vi "总磷总氮通讯.vi"() -> ()   [LabVIEW 2016, in "斯坦道总磷.lvlib"]
uses:
  <vilib>/NI/Modbus Library/API/Wrapper/Create TCP Slave.vi
  <vilib>/Utility/config.llb/Write Key (Boolean).vi
  <vilib>/Utility/config.llb/Write Key (String).vi
  <vilib>/Plasmionique/MB Master/MB_Master/MB_Master.lvclass
  <vilib>/NI/Modbus Library/API/Slave/Modbus Slave.lvclass
  <vilib>/Utility/config.llb/NI_LVConfig.lvlib
  <vilib>/Plasmionique/MB Master/MB Master.lvlib
  <vilib>/NI/Modbus Library/API/Wrapper/API Main.lvlib
  <vilib>/ptbypt/NI_PtbyPt.lvlib
panel:
  out "氨氮状态告警区":u16[](array[numeric])
  out "氨氮测量数据区":u16[](array[numeric])
  out "COD测量数据区":u16[](array[numeric])
  out "COD状态告警区":u16[](array[numeric])
  out "总氮测量数据区":u16[](array[numeric])
  out "总氮状态告警区":u16[](array[numeric])
  out "总磷状态告警区":u16[](array[numeric])
  out "总磷测量数据区":u16[](array[numeric])
  out "状态告警区":T1 {"告警代码" items=["无告警", "缺试剂告警", "缺水样告警", "缺蒸馏水告警", "缺标液告警", "仪表漏液告警", "标定异常告警", "超量程告警", "加热异常", "低试剂预警", "超上限告警", "超下限告警", "仪表内部其他异常", "滴定异常告警", "电极异常告警", "量程切换告警", "参数设置告警", "PH电极电位异常", "电导率电极异常", "浊度光度异常", "溶解氧电极异常", "溶解氧光强异常", "温度异常告警", "PH异常告警", "溶解氧异常告警", "电导率异常告警", "浊度异常告警", "叶绿素异常告警", "藻密度异常告警", "蓝绿藻异常告警", "ORP异常告警", "氨氮异常告警", "清洁刷异常告警", "SD卡异常告警", "蓝牙异常告警", "Wifi异常告警", "流程异常告警"]; "故障代码" items=["无故障", "电机故障", "温度故障", "通讯故障", "滴定故障"]}
  out "测量数据区":T2 {"单位" items=["ug/L", "mg/L", "ppm", "mg/m3", "cm", "ppb", "ug/m3", "%", "nmol/mol", "umol/mol", "MPN/L", "MPN/100ml", "ng/m3", "NTU", "无量纲", "ms/cm", "us/cm", "℃", "mV", "万个/L"]}
  out "status":bool
  out "关键参数区":T3
  in  "读关键参数区":bool
  in  "读状态告警区":bool
  in  "读测量数据区":bool
  in  "站号":u16(ring) items=["总磷"=1, "氨氮"=3]
  in  "停止":bool
  in  "启动":bool
  in  "控制命令":u16(ring) items=["启动测量"=1, "标样核查"=2, "零点核查"=3, "跨度核查"=4, "空白测试"=5, "平行样测试"=6, "加标回收"=7, "空白校准"=8, "标样校准"=9, "初始化（清洗）"=10, "停止测试"=11, "仪器重启"=12, "校时"=13, "模式设置"=14, "测量间隔设置"=15]
  in  "控制命令参数":u16[](array[numeric]) format="%04xH"
  in  "VISA Resource":refnum<visa-resource-name>
  in  "启用模块":bool
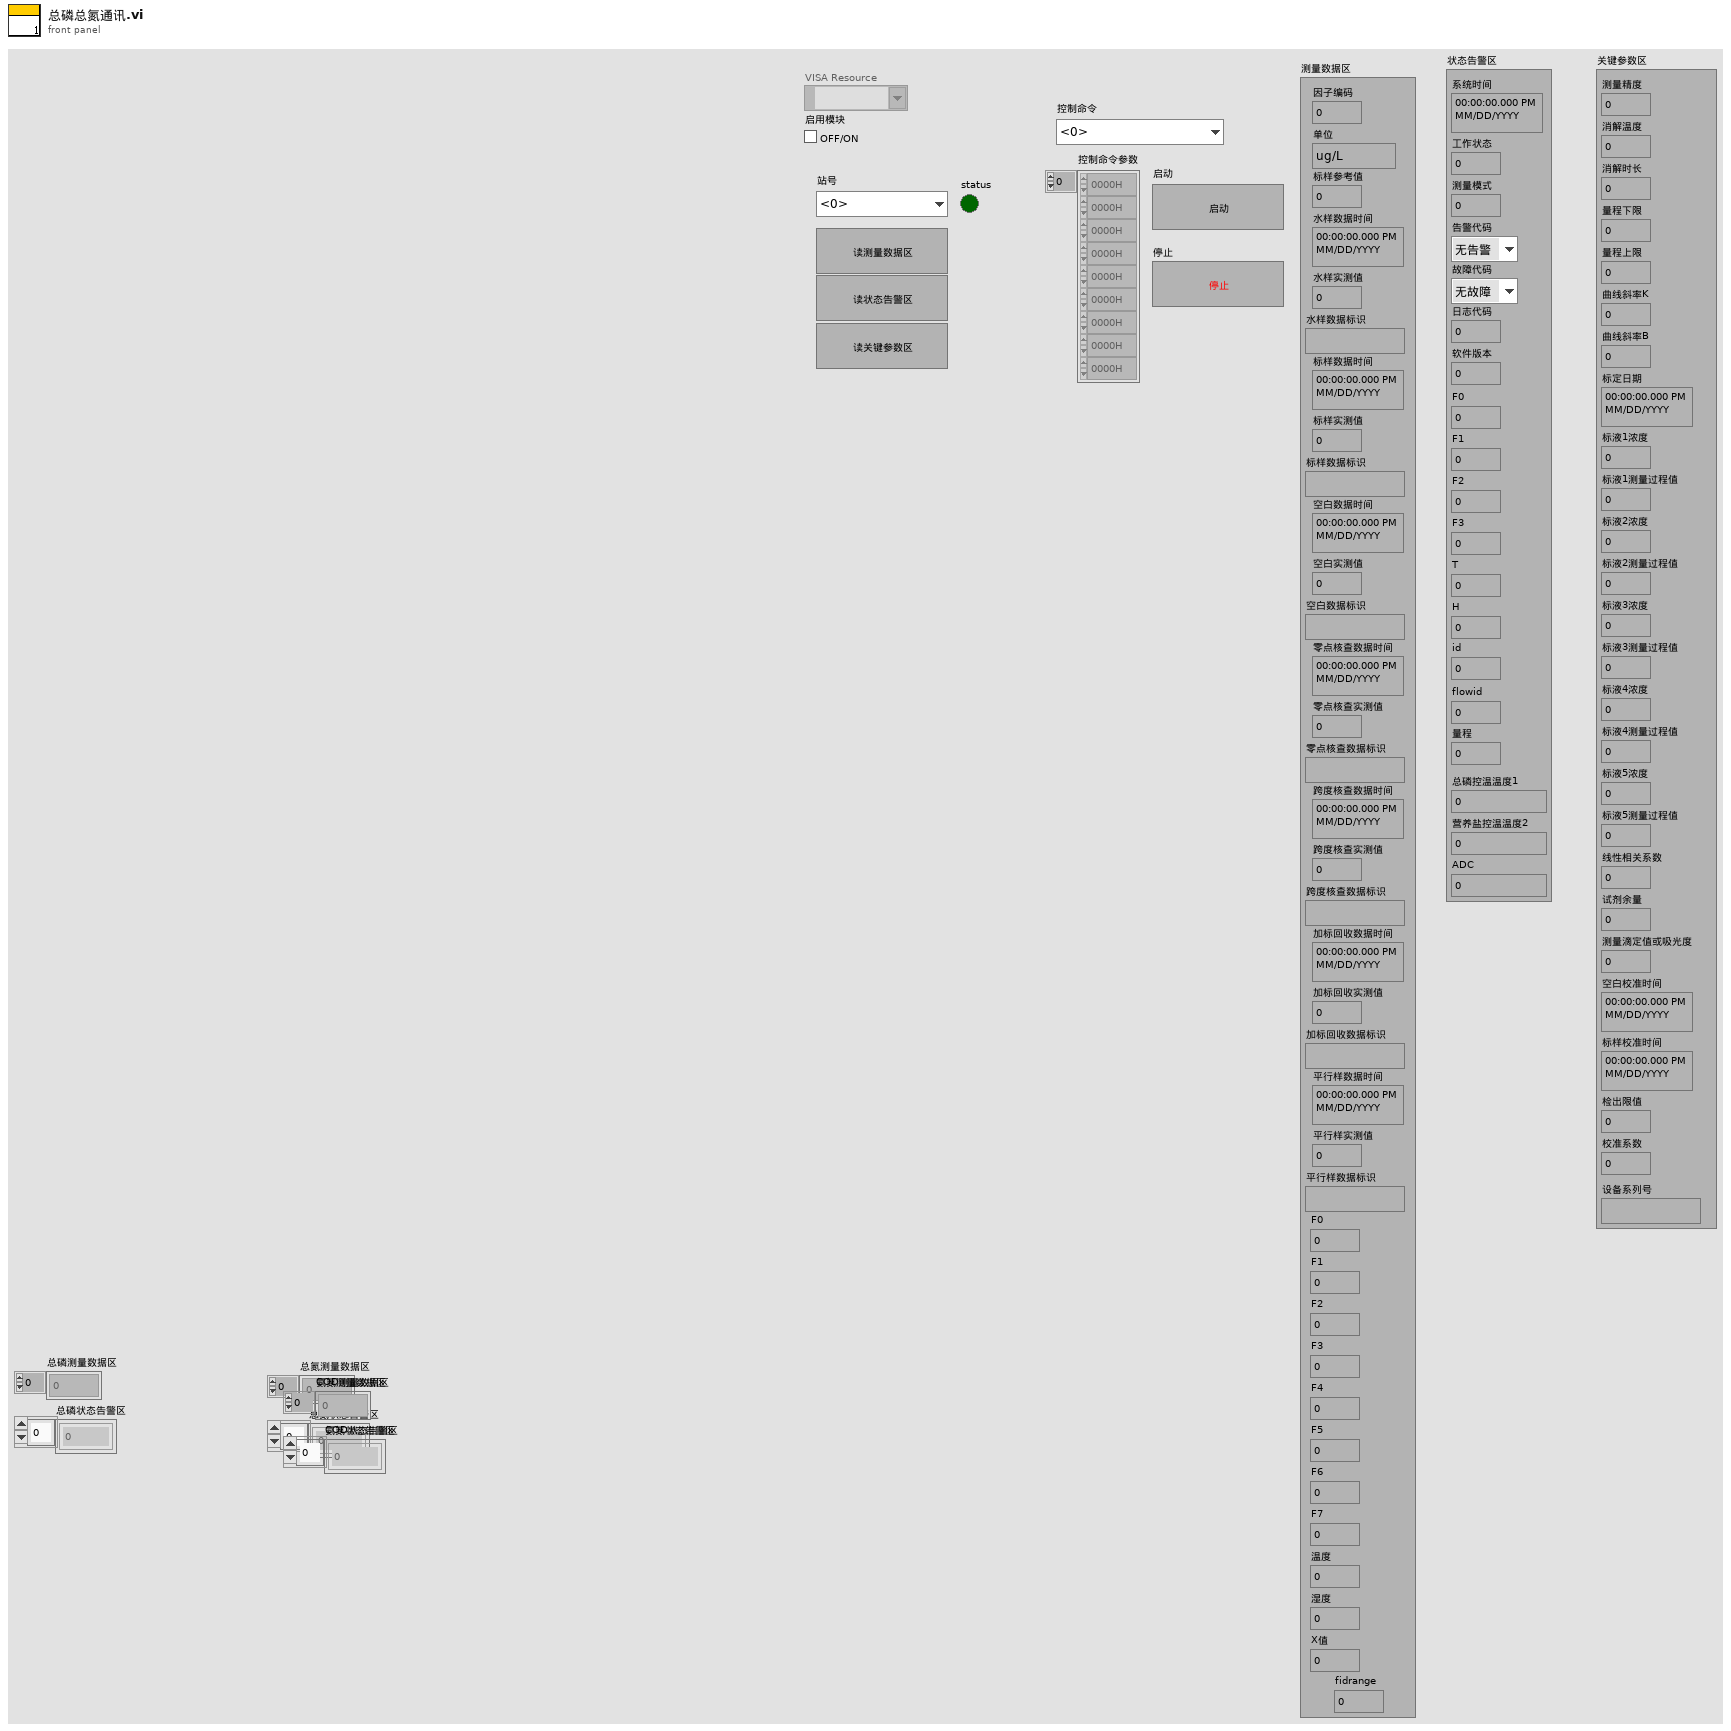
[diagram p1: front panel]
types:
  T1 = cluster{"系统时间":timestamp, "工作状态":u16, "测量模式":u16, "告警代码":u16, "故障代码":u16, "日志代码":u16, "软件版本":u16, "F0":sgl, "F1":sgl, "F2":sgl, "F3":sgl, "T":sgl, "H":sgl, "id":u16, "flowid":u16, "量程":u16, "总磷控温温度1":sgl, "营养盐控温温度2":sgl, "ADC":sgl}
  T2 = cluster{"因子编码":u32, "单位":u16, "标样参考值":sgl, "水样数据时间":timestamp, "水样实测值":sgl, "水样数据标识":string, "标样数据时间":timestamp, "标样实测值":sgl, "标样数据标识":string, "空白数据时间":timestamp, "空白实测值":sgl, "空白数据标识":string, "零点核查数据时间":timestamp, "零点核查实测值":sgl, "零点核查数据标识":string, "跨度核查数据时间":timestamp, "跨度核查实测值":sgl, "跨度核查数据标识":string, "加标回收数据时间":timestamp, "加标回收实测值":sgl, "加标回收数据标识":string, "平行样数据时间":timestamp, "平行样实测值":sgl, "平行样数据标识":string, "F0":sgl, "F1":sgl, "F2":sgl, "F3":sgl, "F4":sgl, "F5":sgl, "F6":sgl, "F7":sgl, "温度":sgl, "湿度":sgl, "X值":sgl, "fidrange":u16}
  T3 = cluster{"测量精度":u16, "消解温度":u16, "消解时长":u16, "量程下限":sgl, "量程上限":sgl, "曲线斜率K":sgl, "曲线斜率B":sgl, "标定日期":timestamp, "标液1浓度":sgl, "标液1测量过程值":sgl, "标液2浓度":sgl, "标液2测量过程值":sgl, "标液3浓度":sgl, "标液3测量过程值":sgl, "标液4浓度":sgl, "标液4测量过程值":sgl, "标液5浓度":sgl, "标液5测量过程值":sgl, "线性相关系数":sgl, "试剂余量":u32, "测量滴定值或吸光度":sgl, "空白校准时间":timestamp, "标样校准时间":timestamp, "检出限值":sgl, "校准系数":sgl, "设备系列号":string}
  T4 = cluster{"系统时间":timestamp, "工作状态":u16, "测量模式":enum16{"待机", "连续模式", "周期模式", "定点模式", "受控模式", "手动模式"}, "告警代码":u16, "故障代码":u16, "日志代码":u16, "软件版本":u16, "F0":sgl, "F1":sgl, "F2":sgl, "F3":sgl, "T":sgl, "H":sgl, "id":u16, "flowid":u16, "量程":u16, "总磷控温温度1":sgl, "营养盐控温温度2":sgl, "ADC":sgl}
  T5 = cluster{"因子编码":u32, "单位":u16, "标样参考值":sgl, "水样数据时间":timestamp, "水样实测值":sgl, "水样数据标识":string, "标样数据时间":timestamp, "标样实测值":sgl, "标样数据标识":string, "空白数据时间":timestamp, "空白实测值":sgl, "空白数据标识":string, "零点核查数据时间":timestamp, "零点核查实测值":sgl, "零点核查数据标识":string, "跨度核查数据时间":timestamp, "跨度核查实测值":sgl, "跨度核查数据标识":string, "加标回收数据时间":timestamp, "加标回收实测值":sgl, "加标回收数据标识":string, "平行样数据时间":timestamp, "平行样实测值":sgl, "平行样数据标识":string, "F0":sgl, "F1":sgl, "F2":sgl, "F3":sgl, "F4":sgl, "F5":sgl, "F6":sgl, "F7":sgl, "温度":sgl, "湿度":sgl, "X值":sgl, "fidrange":u16}[]
  T6 = cluster{"测量精度":u16, "消解温度":u16, "消解时长":u16, "量程下限":sgl, "量程上限":sgl, "曲线斜率K":sgl, "曲线斜率B":sgl, "标定日期":timestamp, "标液1浓度":sgl, "标液1测量过程值":sgl, "标液2浓度":sgl, "标液2测量过程值":sgl, "标液3浓度":sgl, "标液3测量过程值":sgl, "标液4浓度":sgl, "标液4测量过程值":sgl, "标液5浓度":sgl, "标液5测量过程值":sgl, "线性相关系数":sgl, "试剂余量":u32, "测量滴定值或吸光度":sgl, "空白校准时间":timestamp, "标样校准时间":timestamp, "检出限值":sgl, "校准系数":sgl, "设备系列号":string}[]
  T7 = cluster{"系统时间":timestamp, "工作状态":u16, "测量模式":enum16{"待机", "连续模式", "周期模式", "定点模式", "受控模式", "手动模式"}, "告警代码":u16, "故障代码":u16, "日志代码":u16, "软件版本":u16, "F0":sgl, "F1":sgl, "F2":sgl, "F3":sgl, "T":sgl, "H":sgl, "id":u16, "flowid":u16, "量程":u16, "总磷控温温度1":sgl, "营养盐控温温度2":sgl, "ADC":sgl}[]
  T8 = typedef "NI_LVConfig.lvlib/Config Data RefNum.ctl" = refnum<k1>
  T9 = enum8{"Enabled", "Disabled", "Disabled and Grayed Out"}
  T10 = cluster{"时间标识":timestamp, "设备":string, "日志信息":string, "备注":string}
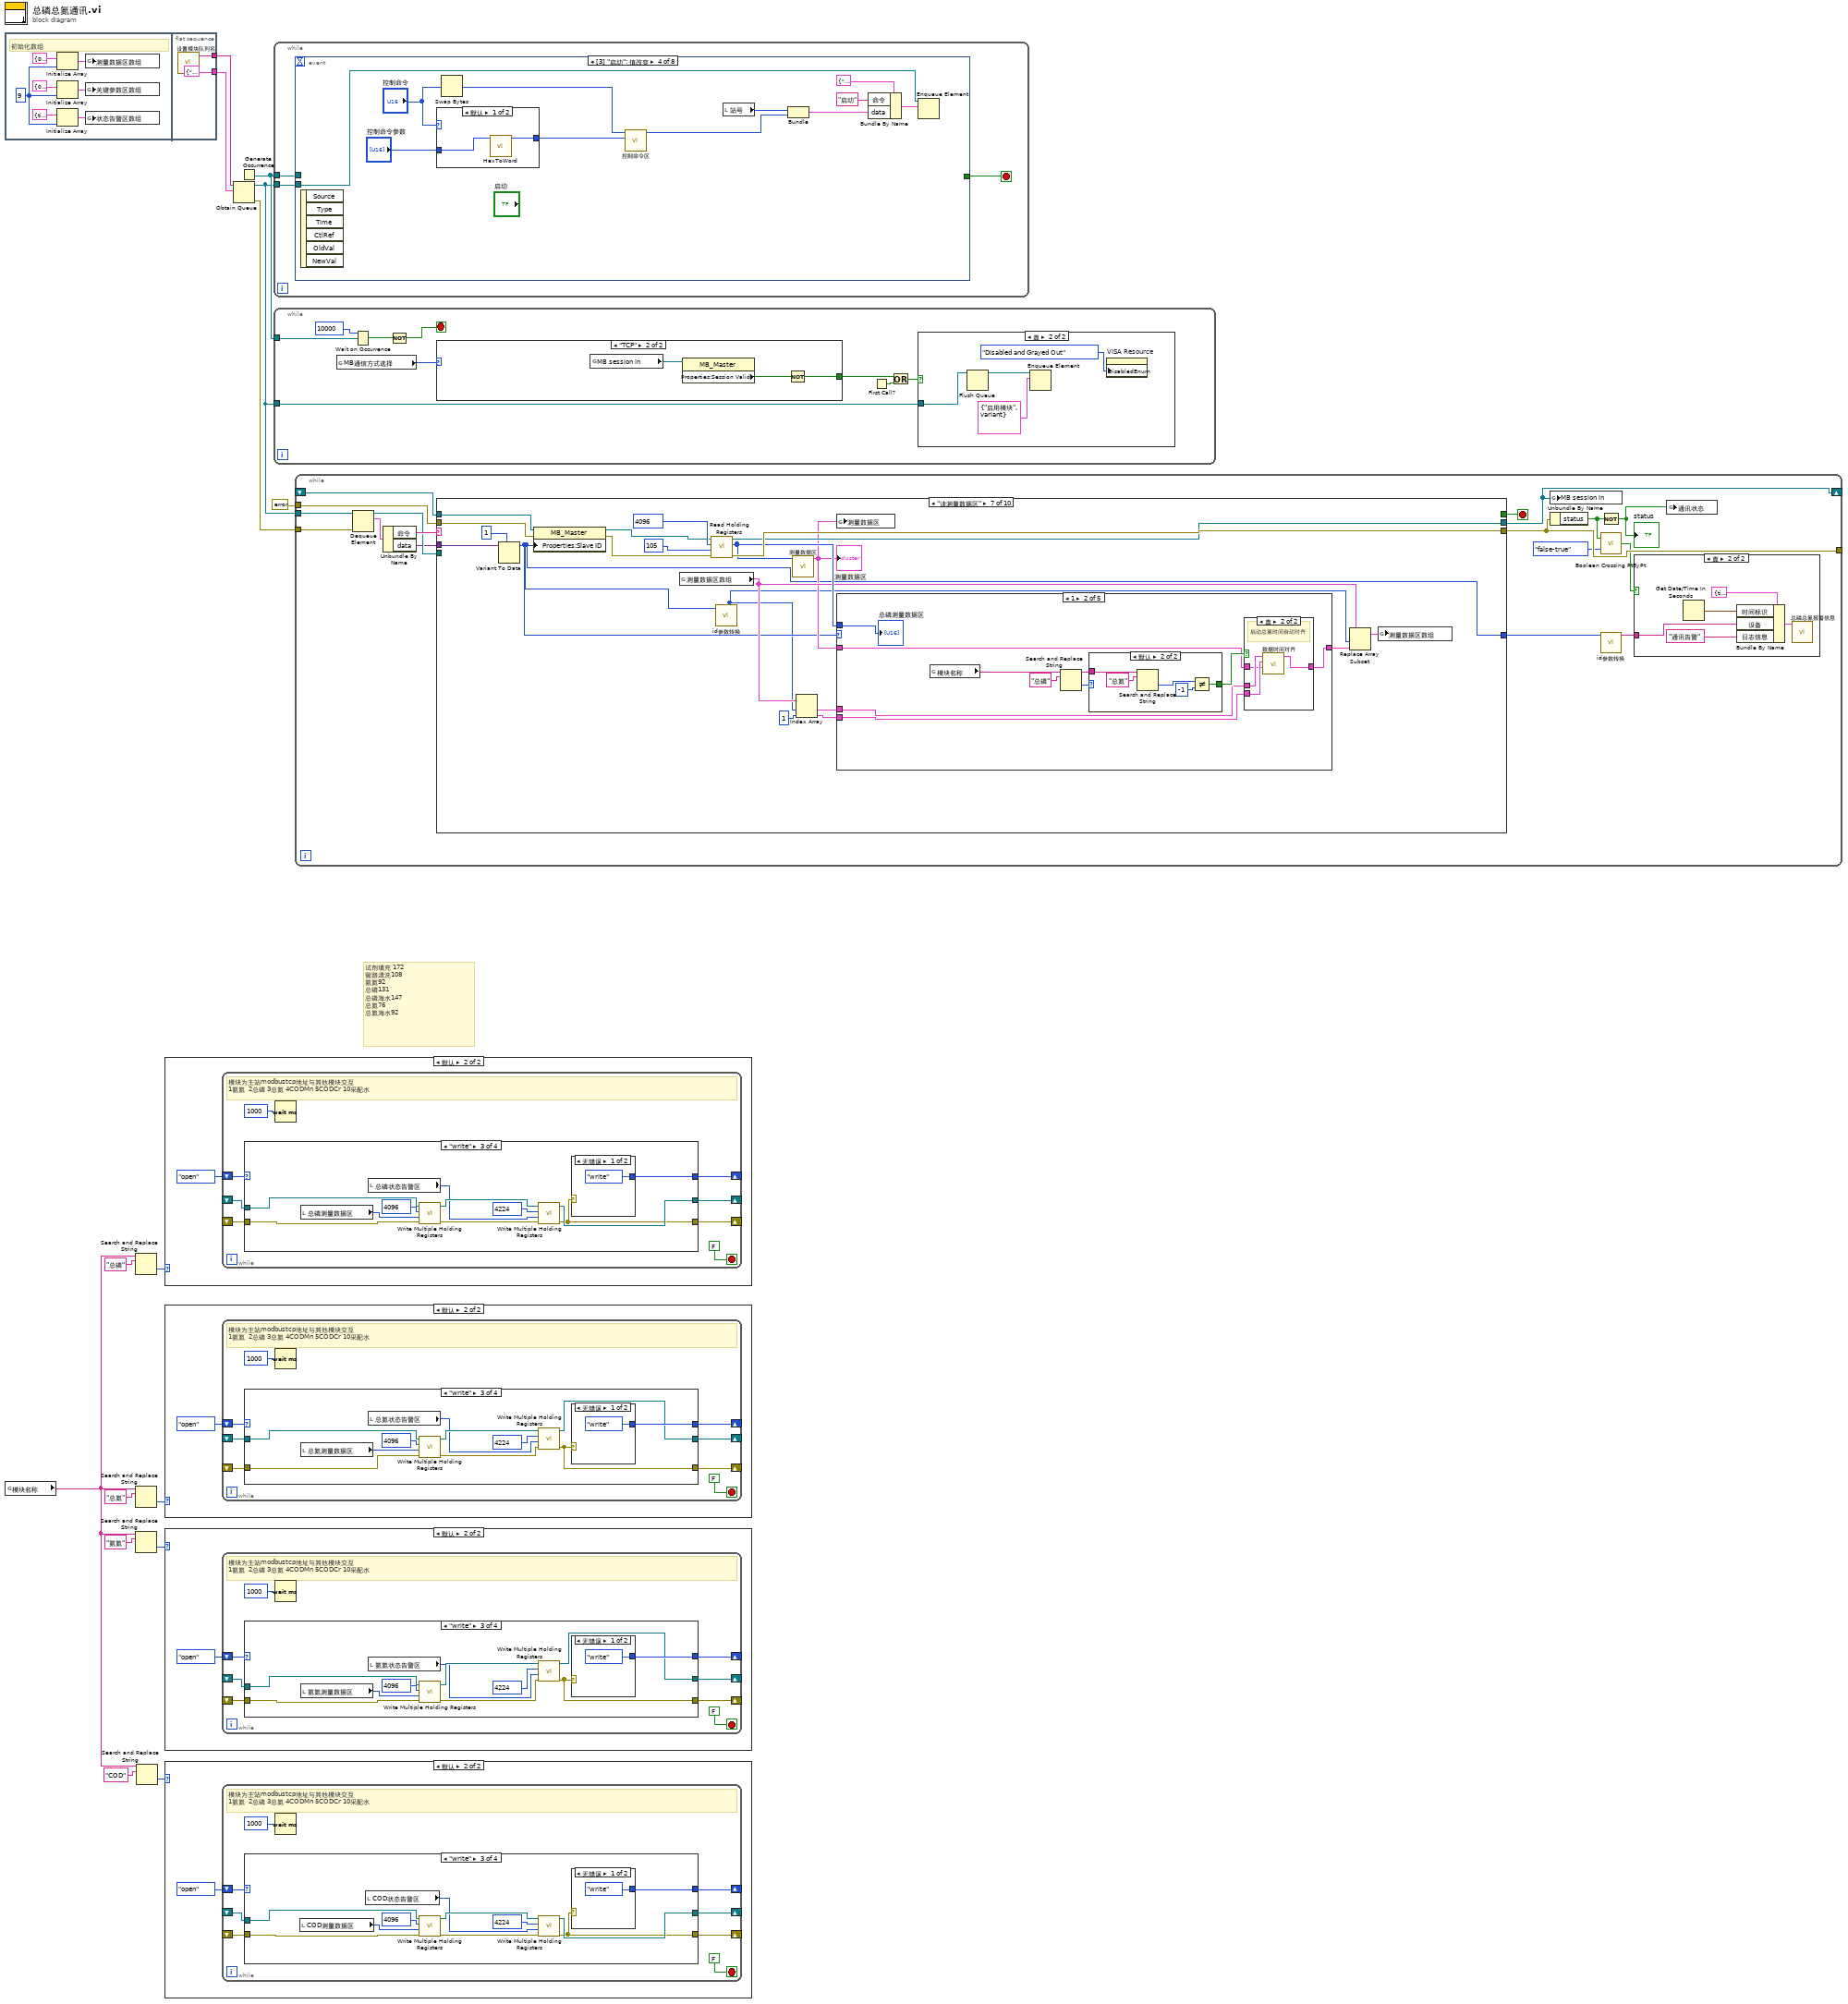
[diagram p0: block diagram]
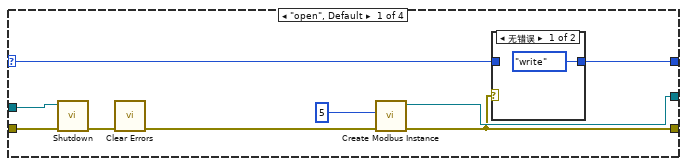
[diagram p3: hidden frame]
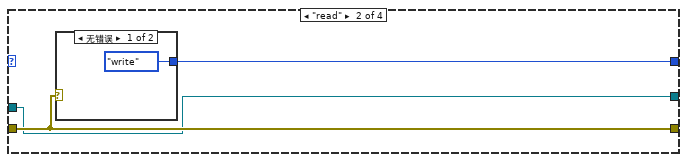
[diagram p5: hidden frame]
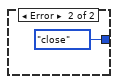
[diagram p6: hidden frame]
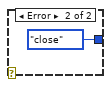
[diagram p7: hidden frame]
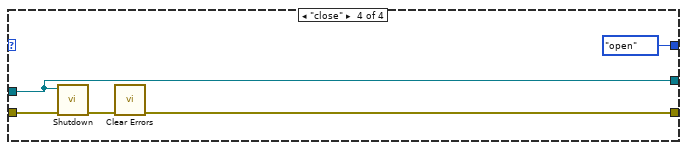
[diagram p8: hidden frame]
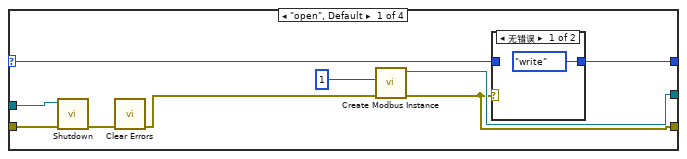
[diagram p10: hidden frame]
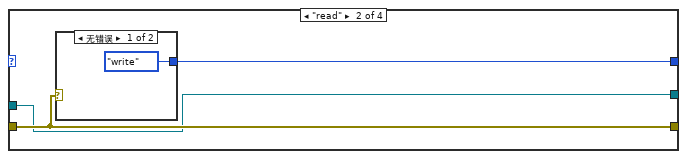
[diagram p12: hidden frame]
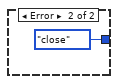
[diagram p13: hidden frame]
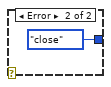
[diagram p14: hidden frame]
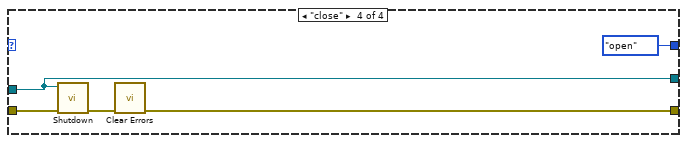
[diagram p15: hidden frame]
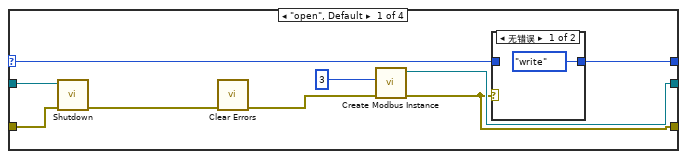
[diagram p17: hidden frame]
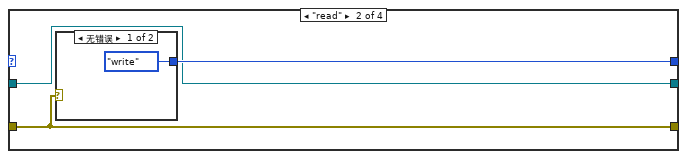
[diagram p19: hidden frame]
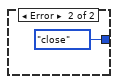
[diagram p20: hidden frame]
diagram:
  # "试剂填充 172 \n管路清洗108\n氨氮92\n总磷131\n总磷海水147\n总氮76\n总氮海水92"
  n1 = flat-sequence {
    tunnel: [cluster{"命令":string, "data":variant} {"命令"="", "data"=variant}] -> w15
    tunnel: [w23] -> w10
    frame #0 {
      w16 = 9 ("维数大小")
      # "初始化数组"
      n2 = Initialize Array(T2 {"因子编码"=0, "单位"=0, "标样参考值"=0.0, "水样数据时间"=timestamp(0 s since 1904-01-01), "水样实测值"=0.0, "水样数据标识"="", "标样数据时间"=timestamp(0 s since 1904-01-01), "标样实测值"=0.0, "标样数据标识"="", "空白数据时间"=timestamp(0 s since 1904-01-01), "空白实测值"=0.0, "空白数据标识"="", "零点核查数据时间"=timestamp(0 s since 1904-01-01), "零点核查实测值"=0.0, "零点核查数据标识"="", "跨度核查数据时间"=timestamp(0 s since 1904-01-01), "跨度核查实测值"=0.0, "跨度核查数据标识"="", "加标回收数据时间"=timestamp(0 s since 1904-01-01), "加标回收实测值"=0.0, "加标回收数据标识"="", "平行样数据时间"=timestamp(0 s since 1904-01-01), "平行样实测值"=0.0, "平行样数据标识"="", "F0"=0.0, "F1"=0.0, "F2"=0.0, "F3"=0.0, "F4"=0.0, "F5"=0.0, "F6"=0.0, "F7"=0.0, "温度"=0.0, "湿度"=0.0, "X值"=0.0, "fidrange"=0} ("测量数据区"), w16) -> (w22:T5)
      n3 = Initialize Array(T3 {"测量精度"=0, "消解温度"=0, "消解时长"=0, "量程下限"=0.0, "量程上限"=0.0, "曲线斜率K"=0.0, "曲线斜率B"=0.0, "标定日期"=timestamp(0 s since 1904-01-01), "标液1浓度"=0.0, "标液1测量过程值"=0.0, "标液2浓度"=0.0, "标液2测量过程值"=0.0, "标液3浓度"=0.0, "标液3测量过程值"=0.0, "标液4浓度"=0.0, "标液4测量过程值"=0.0, "标液5浓度"=0.0, "标液5测量过程值"=0.0, "线性相关系数"=0.0, "试剂余量"=0, "测量滴定值或吸光度"=0.0, "空白校准时间"=timestamp(0 s since 1904-01-01), "标样校准时间"=timestamp(0 s since 1904-01-01), "检出限值"=0.0, "校准系数"=0.0, "设备系列号"=""} ("关键参数区"), w16) -> (w20:T6)
      n4 = Initialize Array(T4 {"系统时间"=timestamp(0 s since 1904-01-01), "工作状态"=0, "测量模式"=enum."待机", "告警代码"=0, "故障代码"=0, "日志代码"=0, "软件版本"=0, "F0"=0.0, "F1"=0.0, "F2"=0.0, "F3"=0.0, "T"=0.0, "H"=0.0, "id"=0, "flowid"=0, "量程"=0, "总磷控温温度1"=0.0, "营养盐控温温度2"=0.0, "ADC"=0.0} ("状态告警区"), w16) -> (w19:T7)
      n5 = global write "VAR总磷总氮全局变量.vi" "测量数据区数组"(w22) -> ()
      n6 = global write "VAR总磷总氮全局变量.vi" "关键参数区数组"(w20) -> ()
      n7 = global write "VAR总磷总氮全局变量.vi" "状态告警区数组"(w19) -> ()
    }
    frame #1 {
      n8 = call "设置模块队列名.vi"() -> ("Msg"=w23:string)  [unwired: 5 in]
    }
  }
  n9 = global read "VAR总磷总氮全局变量.vi" "模块名称"() -> (w3:string)
  n10 = Search and Replace String(input string=w3, search string="总磷" ("搜索字符串")) -> (offset past replacement=w8:i32)  [unwired: 6 in, 3 out]
  n11 = Search and Replace String(input string=w3, search string="总氮" ("搜索字符串")) -> (offset past replacement=w6:i32)  [unwired: 6 in, 3 out]
  n12 = Search and Replace String(input string=w3, search string="氨氮" ("搜索字符串")) -> (offset past replacement=w4:i32)  [unwired: 6 in, 3 out]
  n13 = Search and Replace String(input string=w3, search string="COD" ("搜索字符串")) -> (offset past replacement=w1:i32)  [unwired: 6 in, 3 out]
  n14 = case shown="默认" w8 {
    frame -1 {
    }
    frame Default {
      n15 = while {
        shift-right: [w31] -> _
        shift-left: _ -> [w33]
        shift-right: [w30] -> _
        shift-left: _ -> [w32]
        shift-right: [w27] -> _
        shift-left: enum16{"open", "read", "write", "close"}."open" -> [w28]
        stop <- FALSE stop-if-true
        # "模块为主站modbustcp地址与其他模块交互\n1氨氮  2总磷 3总氮 4CODMn 5CODCr 10采配水"
        n16 = case shown="\"write\"" w28 {
          selector: w28 -> [w42 _ _ _]
          tunnel: w33 -> [w36 w45 w51 w65]
          tunnel: w32 -> [w35 w46 w50 w64]
          tunnel: [w39 w45 w56 w65] -> w31
          tunnel: [w38 w46 w55 w67] -> w30
          tunnel: [w41 w47 w60 enum16{"open", "read", "write", "close"}."open"] -> w27
          frame "open", Default {
            n17 = call-dynamic "Shutdown.vi"("error in"=w35, "Modbus slave in"=w36) -> ("error out"=w34:errorcluster)  [unwired: 9 in]
            n18 = call <vilib>:"Clear Errors.vi"("error in (no error)"=w34) -> ("error out"=w37:errorcluster)  [unwired: 5 in, 1 out]
            n19 = call-poly <vilib>:"Create Modbus Instance.vi"("error in"=w37, "port (502)"=u16 2) -> ("error out"=w38:errorcluster, "TCP slave instance"=w39:refnum<class "Modbus Slave.lvclass">)  [unwired: 8 in]
            n20 = case shown="无错误" w38 {
              tunnel: w42 -> [_ w44]
              tunnel: [enum16{"open", "read", "write", "close"}."write" w44] -> w41
              frame No Error {
              }
              frame Error {
              }
            }
          }
          frame "read" {
            n21 = case shown="无错误" w46 {
              tunnel: [enum16{"open", "read", "write", "close"}."write" enum16{"open", "read", "write", "close"}."close"] -> w47
              frame No Error {
              }
              frame Error {
              }
            }
          }
          frame "write" {
            n22 = local read "总磷测量数据区"() -> (w54:u16[])
            n23 = local read "总磷状态告警区"() -> (w52:u16[])
            n24 = call-dynamic "Write Multiple Holding Registers.vi"("error in"=w50, "registers to write"=w54, "starting address"=u16 4096, "Modbus slave in"=w51) -> ("error out"=w57:errorcluster, "Modbus slave out"=w58:refnum<class "Modbus Slave.lvclass">)  [unwired: 6 in]
            n25 = call-dynamic "Write Multiple Holding Registers.vi"("error in"=w57, "registers to write"=w52, "starting address"=u16 4224, "Modbus slave in"=w58) -> ("error out"=w55:errorcluster, "Modbus slave out"=w56:refnum<class "Modbus Slave.lvclass">)  [unwired: 6 in]
            n26 = case shown="无错误" w55 {
              tunnel: [enum16{"open", "read", "write", "close"}."write" enum16{"open", "read", "write", "close"}."close"] -> w60
              frame No Error {
              }
              frame Error {
              }
            }
          }
          frame "close" {
            n27 = call-dynamic "Shutdown.vi"("error in"=w64, "Modbus slave in"=w65) -> ("error out"=w63:errorcluster)  [unwired: 9 in]
            n28 = call <vilib>:"Clear Errors.vi"("error in (no error)"=w63) -> ("error out"=w67:errorcluster)  [unwired: 5 in, 1 out]
          }
        }
        n29 = Wait (ms)(milliseconds to wait=u32 1000 ("等待时间（毫秒）")) -> ()  [unwired: 1 out]
      }
    }
  }
  n30 = case shown="默认" w6 {
    frame -1 {
    }
    frame Default {
      n31 = while {
        shift-right: [w74] -> _
        shift-left: _ -> [w76]
        shift-right: [w73] -> _
        shift-left: _ -> [w75]
        shift-right: [w70] -> _
        shift-left: enum16{"open", "read", "write", "close"}."open" -> [w71]
        stop <- FALSE stop-if-true
        # "模块为主站modbustcp地址与其他模块交互\n1氨氮  2总磷 3总氮 4CODMn 5CODCr 10采配水"
        n32 = case shown="\"write\"" w71 {
          selector: w71 -> [w85 _ _ _]
          tunnel: w76 -> [w79 w88 w94 w108]
          tunnel: w75 -> [w78 w89 w93 w107]
          tunnel: [w82 w88 w99 w108] -> w74
          tunnel: [w81 w89 w98 w110] -> w73
          tunnel: [w84 w90 w103 enum16{"open", "read", "write", "close"}."open"] -> w70
          frame "open", Default {
            n33 = call-dynamic "Shutdown.vi"("error in"=w78, "Modbus slave in"=w79) -> ("error out"=w77:errorcluster)  [unwired: 9 in]
            n34 = call <vilib>:"Clear Errors.vi"("error in (no error)"=w77) -> ("error out"=w80:errorcluster)  [unwired: 5 in, 1 out]
            n35 = call-poly <vilib>:"Create Modbus Instance.vi"("error in"=w80, "port (502)"=u16 3) -> ("error out"=w81:errorcluster, "TCP slave instance"=w82:refnum<class "Modbus Slave.lvclass">)  [unwired: 8 in]
            n36 = case shown="无错误" w81 {
              tunnel: w85 -> [_ w87]
              tunnel: [enum16{"open", "read", "write", "close"}."write" w87] -> w84
              frame No Error {
              }
              frame Error {
              }
            }
          }
          frame "read" {
            n37 = case shown="无错误" w89 {
              tunnel: [enum16{"open", "read", "write", "close"}."write" enum16{"open", "read", "write", "close"}."close"] -> w90
              frame No Error {
              }
              frame Error {
              }
            }
          }
          frame "write" {
            n38 = local read "总氮测量数据区"() -> (w97:u16[])
            n39 = local read "总氮状态告警区"() -> (w95:u16[])
            n40 = call-dynamic "Write Multiple Holding Registers.vi"("error in"=w93, "registers to write"=w97, "starting address"=u16 4096, "Modbus slave in"=w94) -> ("error out"=w100:errorcluster, "Modbus slave out"=w101:refnum<class "Modbus Slave.lvclass">)  [unwired: 6 in]
            n41 = call-dynamic "Write Multiple Holding Registers.vi"("error in"=w100, "registers to write"=w95, "starting address"=u16 4224, "Modbus slave in"=w101) -> ("error out"=w98:errorcluster, "Modbus slave out"=w99:refnum<class "Modbus Slave.lvclass">)  [unwired: 6 in]
            n42 = case shown="无错误" w98 {
              tunnel: [enum16{"open", "read", "write", "close"}."write" enum16{"open", "read", "write", "close"}."close"] -> w103
              frame No Error {
              }
              frame Error {
              }
            }
          }
          frame "close" {
            n43 = call-dynamic "Shutdown.vi"("error in"=w107, "Modbus slave in"=w108) -> ("error out"=w106:errorcluster)  [unwired: 9 in]
            n44 = call <vilib>:"Clear Errors.vi"("error in (no error)"=w106) -> ("error out"=w110:errorcluster)  [unwired: 5 in, 1 out]
          }
        }
        n45 = Wait (ms)(milliseconds to wait=u32 1000 ("等待时间（毫秒）")) -> ()  [unwired: 1 out]
      }
    }
  }
  n46 = case shown="默认" w4 {
    frame -1 {
    }
    frame Default {
      n47 = while {
        shift-right: [w117] -> _
        shift-left: _ -> [w119]
        shift-right: [w116] -> _
        shift-left: _ -> [w118]
        shift-right: [w113] -> _
        shift-left: enum16{"open", "read", "write", "close"}."open" -> [w114]
        stop <- FALSE stop-if-true
        # "模块为主站modbustcp地址与其他模块交互\n1氨氮  2总磷 3总氮 4CODMn 5CODCr 10采配水"
        n48 = case shown="\"write\"" w114 {
          selector: w114 -> [w128 _ _ _]
          tunnel: w119 -> [w122 w131 w137 w151]
          tunnel: w118 -> [w121 w132 w136 w150]
          tunnel: [w125 w131 w142 w151] -> w117
          tunnel: [w124 w132 w141 w153] -> w116
          tunnel: [w127 w133 w146 enum16{"open", "read", "write", "close"}."open"] -> w113
          frame "open", Default {
            n49 = call-dynamic "Shutdown.vi"("error in"=w121, "Modbus slave in"=w122) -> ("error out"=w120:errorcluster)  [unwired: 9 in]
            n50 = call <vilib>:"Clear Errors.vi"("error in (no error)"=w120) -> ("error out"=w123:errorcluster)  [unwired: 5 in, 1 out]
            n51 = call-poly <vilib>:"Create Modbus Instance.vi"("error in"=w123, "port (502)"=u16 1) -> ("error out"=w124:errorcluster, "TCP slave instance"=w125:refnum<class "Modbus Slave.lvclass">)  [unwired: 8 in]
            n52 = case shown="无错误" w124 {
              tunnel: w128 -> [_ w130]
              tunnel: [enum16{"open", "read", "write", "close"}."write" w130] -> w127
              frame No Error {
              }
              frame Error {
              }
            }
          }
          frame "read" {
            n53 = case shown="无错误" w132 {
              tunnel: [enum16{"open", "read", "write", "close"}."write" enum16{"open", "read", "write", "close"}."close"] -> w133
              frame No Error {
              }
              frame Error {
              }
            }
          }
          frame "write" {
            n54 = local read "氨氮测量数据区"() -> (w140:u16[])
            n55 = local read "氨氮状态告警区"() -> (w138:u16[])
            n56 = call-dynamic "Write Multiple Holding Registers.vi"("error in"=w136, "registers to write"=w140, "starting address"=u16 4096, "Modbus slave in"=w137) -> ("error out"=w143:errorcluster, "Modbus slave out"=w144:refnum<class "Modbus Slave.lvclass">)  [unwired: 6 in]
            n57 = call-dynamic "Write Multiple Holding Registers.vi"("error in"=w143, "registers to write"=w138, "starting address"=u16 4224, "Modbus slave in"=w144) -> ("error out"=w141:errorcluster, "Modbus slave out"=w142:refnum<class "Modbus Slave.lvclass">)  [unwired: 6 in]
            n58 = case shown="无错误" w141 {
              tunnel: [enum16{"open", "read", "write", "close"}."write" enum16{"open", "read", "write", "close"}."close"] -> w146
              frame No Error {
              }
              frame Error {
              }
            }
          }
          frame "close" {
            n59 = call-dynamic "Shutdown.vi"("error in"=w150, "Modbus slave in"=w151) -> ("error out"=w149:errorcluster)  [unwired: 9 in]
            n60 = call <vilib>:"Clear Errors.vi"("error in (no error)"=w149) -> ("error out"=w153:errorcluster)  [unwired: 5 in, 1 out]
          }
        }
        n61 = Wait (ms)(milliseconds to wait=u32 1000 ("等待时间（毫秒）")) -> ()  [unwired: 1 out]
      }
    }
  }
  n62 = case shown="默认" w1 {
    frame -1 {
    }
    frame Default {
      n63 = while {
        shift-right: [w160] -> _
        shift-left: _ -> [w162]
        shift-right: [w159] -> _
        shift-left: _ -> [w161]
        shift-right: [w156] -> _
        shift-left: enum16{"open", "read", "write", "close"}."open" -> [w157]
        stop <- FALSE stop-if-true
        # "模块为主站modbustcp地址与其他模块交互\n1氨氮  2总磷 3总氮 4CODMn 5CODCr 10采配水"
        n64 = case shown="\"write\"" w157 {
          selector: w157 -> [w171 _ _ _]
          tunnel: w162 -> [w165 w174 w180 w194]
          tunnel: w161 -> [w164 w175 w179 w193]
          tunnel: [w168 w174 w185 w194] -> w160
          tunnel: [w167 w175 w184 w196] -> w159
          tunnel: [w170 w176 w189 enum16{"open", "read", "write", "close"}."open"] -> w156
          frame "open", Default {
            n65 = call-dynamic "Shutdown.vi"("error in"=w164, "Modbus slave in"=w165) -> ("error out"=w163:errorcluster)  [unwired: 9 in]
            n66 = call <vilib>:"Clear Errors.vi"("error in (no error)"=w163) -> ("error out"=w166:errorcluster)  [unwired: 5 in, 1 out]
            n67 = call-poly <vilib>:"Create Modbus Instance.vi"("error in"=w166, "port (502)"=u16 5) -> ("error out"=w167:errorcluster, "TCP slave instance"=w168:refnum<class "Modbus Slave.lvclass">)  [unwired: 8 in]
            n68 = case shown="无错误" w167 {
              tunnel: w171 -> [_ w173]
              tunnel: [enum16{"open", "read", "write", "close"}."write" w173] -> w170
              frame No Error {
              }
              frame Error {
              }
            }
          }
          frame "read" {
            n69 = case shown="无错误" w175 {
              tunnel: [enum16{"open", "read", "write", "close"}."write" enum16{"open", "read", "write", "close"}."close"] -> w176
              frame No Error {
              }
              frame Error {
              }
            }
          }
          frame "write" {
            n70 = local read "COD测量数据区"() -> (w183:u16[])
            n71 = local read "COD状态告警区"() -> (w181:u16[])
            n72 = call-dynamic "Write Multiple Holding Registers.vi"("error in"=w179, "registers to write"=w183, "starting address"=u16 4096, "Modbus slave in"=w180) -> ("error out"=w186:errorcluster, "Modbus slave out"=w187:refnum<class "Modbus Slave.lvclass">)  [unwired: 6 in]
            n73 = call-dynamic "Write Multiple Holding Registers.vi"("error in"=w186, "registers to write"=w181, "starting address"=u16 4224, "Modbus slave in"=w187) -> ("error out"=w184:errorcluster, "Modbus slave out"=w185:refnum<class "Modbus Slave.lvclass">)  [unwired: 6 in]
            n74 = case shown="无错误" w184 {
              tunnel: [enum16{"open", "read", "write", "close"}."write" enum16{"open", "read", "write", "close"}."close"] -> w189
              frame No Error {
              }
              frame Error {
              }
            }
          }
          frame "close" {
            n75 = call-dynamic "Shutdown.vi"("error in"=w193, "Modbus slave in"=w194) -> ("error out"=w192:errorcluster)  [unwired: 9 in]
            n76 = call <vilib>:"Clear Errors.vi"("error in (no error)"=w192) -> ("error out"=w196:errorcluster)  [unwired: 5 in, 1 out]
          }
        }
        n77 = Wait (ms)(milliseconds to wait=u32 1000 ("等待时间（毫秒）")) -> ()  [unwired: 1 out]
      }
    }
  }
  n78 = Obtain Queue(name (unnamed)=w10, element data type=w15) -> (queue out=w11:refnum<queue>, error out=w14:errorcluster)  [unwired: 3 in, 1 out]
  n79 = Generate Occurrence() -> (w12:refnum<k4>)
  n80 = while {
    tunnel: w11 -> [w199]
    tunnel: w12 -> [w197]
    stop <- w198 stop-if-true
    n81 = event shown="[3] \"启动\": 值改变" {
      selector: _ -> [_ _ _ _ _ _ _ _]
      dyn-events: _ -> [_ _ _ _ _ _ _ _]
      timeout: _ -> [_ _ _ _ _ _ _ _]
      tunnel: w199 -> [_ _ _ w230 w237 w243 w248 w253]
      tunnel: [_ _ _ _ "停止" _ _ _] -> w198
      tunnel: w197 -> [_ _ _ _ w234 _ _ _]
      event Timeout {
        n82 = event-data() -> ()  [unwired: 1 in, 3 out]
      }
      event "启用模块": Value Change {
        n83 = event-data() -> ("NewVal"=w200:bool)  [unwired: 1 in, 5 out]
        n84 = call <vilib>:"Application Directory.vi"() -> ("Application Directory"=w202:path)
        n85 = Build Path(base path=w202, name or relative path="data\\set.ini" ("名称或相对路径")) -> (appended path=w203:path)
        n86 = call <vilib>:"Open Config Data.vi"("configuration file path"=w203) -> ("error out"=w209:errorcluster, "refnum"=w208:T8)  [unwired: 8 in, 1 out]
        n87 = call-poly <vilib>:"Write Key.vi"("section"="总磷总氮", "error in (no error)"=w209, "value"=w200, "key"="模块启用", "refnum"=w208) -> ("error out"=w205:errorcluster, "refnum out"=w201:T8)  [unwired: 4 in, 1 out]
        n88 = call <vilib>:"Close Config Data.vi"("error in (no error)"=w205, "refnum"=w201) -> ()  [unwired: 8 in, 2 out]
      }
      event "VISA Resource": Value Change {
        n89 = event-data() -> ()  [unwired: 1 in, 6 out]
        n90 = call <vilib>:"Application Directory.vi"() -> ("Application Directory"=w212:path)
        n91 = Build Path(base path=w212, name or relative path="data\\set.ini" ("名称或相对路径")) -> (appended path=w213:path)
        n92 = call <vilib>:"Open Config Data.vi"("configuration file path"=w213) -> ("error out"=w219:errorcluster, "refnum"=w218:T8)  [unwired: 8 in, 1 out]
        n93 = call-poly <vilib>:"Write Key.vi"("section"="总磷总氮", "error in (no error)"=w219, "value"="VISA Resource", "key"="串口", "refnum"=w218) -> ("error out"=w215:errorcluster, "refnum out"=w211:T8)  [unwired: 4 in, 1 out]
        n94 = call <vilib>:"Close Config Data.vi"("error in (no error)"=w215, "refnum"=w211) -> ()  [unwired: 8 in, 2 out]
      }
      event "启动": Value Change {
        n95 = event-data() -> ()  [unwired: 1 in, 6 out]
        n96 = case shown="默认" "控制命令" {
          tunnel: "控制命令参数" -> [w232 w233]
          tunnel: [w231 w233] -> w220
          frame Default {
            n97 = call "HexToWord.vi"("数组"=w232) -> ("WORD"=w231:u16[])  [unwired: 10 in]
          }
          frame 13 {
          }
        }
        n98 = Swap Bytes(anything="控制命令") -> (byte swapped=w223:u16)
        n99 = call "控制命令区.vi"("控制命令参数"=w220, "控制命令"=w223) -> ("控制命令"=w226:u16[])  [unwired: 9 in]
        n100 = local read "站号"() -> (w225:u16)
        n101 = Bundle("站号"=w225, "控制命令"=w226) -> (w224:cluster{"站号":u16, "控制命令":u16[]})  [unwired: 1 in]
        n102 = Bundle By Name(cluster=cluster{"命令":string, "data":variant} {"命令"="", "data"=variant} ("元素"), "命令"="启动", "data"=w224) -> (w228:cluster{"命令":string, "data":variant})
        n103 = Enqueue Element(queue=w230, element=w228) -> ()  [unwired: 2 in, 3 out]
      }
      event "停止": Value Change {
        n104 = event-data() -> ()  [unwired: 1 in, 6 out]
        n105 = Set Occurrence(w234) -> ()
        n106 = Flush Queue(queue=w237) -> (queue out=w236:refnum<queue>)  [unwired: 1 in, 2 out]
        n107 = Enqueue Element(queue=w236, element=cluster{"命令":string, "data":variant} {"命令"="shutdown", "data"=variant} ("元素")) -> ()  [unwired: 2 in, 3 out]
      }
      event "读测量数据区": Value Change {
        n108 = event-data() -> ()  [unwired: 1 in, 6 out]
        n109 = Bundle By Name(cluster=cluster{"命令":string, "data":variant} {"命令"="", "data"=variant} ("元素"), "命令"="读测量数据区", "data"="站号") -> (w241:cluster{"命令":string, "data":variant})
        n110 = Enqueue Element(queue=w243, element=w241) -> ()  [unwired: 2 in, 3 out]
      }
      event "读状态告警区": Value Change {
        n111 = event-data() -> ()  [unwired: 1 in, 6 out]
        n112 = local read "站号"() -> (w244:u16)
        n113 = Bundle By Name(cluster=cluster{"命令":string, "data":variant} {"命令"="", "data"=variant} ("元素"), "命令"="读状态告警区", "data"=w244) -> (w246:cluster{"命令":string, "data":variant})
        n114 = Enqueue Element(queue=w248, element=w246) -> ()  [unwired: 2 in, 3 out]
      }
      event "读关键参数区": Value Change {
        n115 = event-data() -> ()  [unwired: 1 in, 6 out]
        n116 = local read "站号"() -> (w249:u16)
        n117 = Bundle By Name(cluster=cluster{"命令":string, "data":variant} {"命令"="", "data"=variant} ("元素"), "命令"="读关键参数区", "data"=w249) -> (w251:cluster{"命令":string, "data":variant})
        n118 = Enqueue Element(queue=w253, element=w251) -> ()  [unwired: 2 in, 3 out]
      }
    }
  }
  n119 = while {
    tunnel: w12 -> [w262]
    tunnel: w11 -> [w258]
    stop <- w259 stop-if-true
    n120 = global read "总磷总氮断电保存全局变量.vi" "MB通信方式选择"() -> (w257:enum16{"串口", "TCP"})
    n121 = Wait on Occurrence(2:w262, 3:10000 ("毫秒超时(-1)")) -> (0:w260:bool)  [unwired: 1 in]
    n122 = Not(x=w260) -> (.not. x?=w259:bool)
    n123 = case shown="\"TCP\"" w257 {
      tunnel: [_ w263] -> w254
      frame "串口", Default {
      }
      frame "TCP" {
        n124 = global read "VAR总磷总氮全局变量.vi" "MB session in"() -> (w265:refnum<class "MB_Master.lvclass">)
        n125 = property class="MB_Master"(reference=w265) -> ("Properties:Session Valid"=w264:bool)  [unwired: 1 in, 2 out]
        n126 = Not(x=w264) -> (.not. x?=w263:bool)
      }
    }
    n127 = First Call?() -> (First Call?: T/F=w256:bool)
    n128 = Or(x=w254, y=w256) -> (x .or. y?=w255:bool)
    n129 = case shown="真" w255 {
      tunnel: w258 -> [_ w268]
      frame False {
      }
      frame True {
        n130 = Flush Queue(queue=w268) -> (queue out=w266:refnum<queue>)  [unwired: 1 in, 2 out]
        n131 = Enqueue Element(queue=w266, element=cluster{"命令":string, "data":variant} {"命令"="启用模块", "data"=variant} ("元素")) -> ()  [unwired: 2 in, 3 out]
        n132 = property on="VISA Resource" class="VISAName"("DisabledEnum"=T9."Disabled and Grayed Out" ("禁用")) -> ()  [unwired: 2 in, 2 out]
      }
    }
  }
  n133 = while {
    tunnel: w11 -> [w286]
    tunnel: w14 -> [w285]
    shift-right: [w270] -> _
    shift-left: _ -> [w283]
    tunnel: errorcluster {"status"=FALSE, "code"=0, "source"=""} ("error out") -> [w282]
    tunnel: [w278] -> _
    stop <- w284 stop-if-true
    n134 = Dequeue Element(queue=w286, error in (no error)=w285) -> (queue out=w279:refnum<queue>, element=w280:cluster{"命令":string, "data":variant})  [unwired: 1 in, 2 out]
    n135 = Unbundle By Name(w280) -> ("命令"=w281:string, "data"=w276:variant)
    n136 = case shown="\"读测量数据区\"" w281 {
      tunnel: w276 -> [_ _ _ w313 w324 w341 w358 w399 w419 _]
      tunnel: w279 -> [_ _ _ _ _ _ _ _ _ w432]
      tunnel: [_ _ _ _ _ _ _ _ _ TRUE] -> w284
      tunnel: [w292 w294 w300 w316 w327 w343 w362 w407 w426 w428] -> w270
      tunnel: [w293 w295 w301 w315 w326 w342 w363 w398 w427 w429] -> w278
      tunnel: w283 -> [w292 _ w300 w312 w323 w340 w357 w402 w422 w428]
      tunnel: w282 -> [w293 _ w302 w309 w320 w337 w355 w403 w423 w430]
      tunnel: [_ _ _ w304 w317 w331 w345 w392 w413 _] -> w271
      frame Default {
      }
      frame "启用模块" {
        n137 = call "总磷总氮MB_api.vi"("STEP"=enum16{"open", "read", "write", "close"}."open") -> ("error out"=w295:errorcluster, "MB session out"=w294:refnum<class "MB_Master.lvclass">)  [unwired: 8 in, 1 out]
      }
      frame "停用模块" {
        n138 = call-dynamic "Close Session.vi"("error in (no error)"=w302, "MB session in"=w300) -> ("error out"=w299:errorcluster)  [unwired: 9 in]
        n139 = call "总磷总氮MB_api.vi"("STEP"=enum16{"open", "read", "write", "close"}."close", "Error in"=w299) -> ("error out"=w298:errorcluster)  [unwired: 7 in, 2 out]
        n140 = call <vilib>:"Clear Errors.vi"("error in (no error)"=w298) -> ("error out"=w301:errorcluster)  [unwired: 5 in, 1 out]
      }
      frame "启动" {
        n141 = Variant To Data(type=cluster{"站号":u16, "控制命令":u16[]} {"站号"=0, "控制命令"=[]} ("输出簇"), Variant=w313) -> (data=w307:cluster{"站号":u16, "控制命令":u16[]})  [unwired: 1 in, 1 out]
        n142 = Unbundle By Name(w307) -> ("站号"=w304:u16, "控制命令"=w305:u16[])
        n143 = property class="MB_Master"(reference=w312, error in=w309, "Properties:Slave ID"=w304) -> (reference out=w311:refnum<class "MB_Master.lvclass">, error out=w310:errorcluster)
        n144 = Index Array(array=w305) -> (element=w306:u16)  [unwired: 1 in]
        n145 = Swap Bytes(anything=w306) -> (byte swapped=w303:u16)
        n146 = global write "VAR总磷总氮全局变量.vi" "控制命令"(w303) -> ()
        n147 = call <vilib>:"Write Multiple Registers.vi"("error in (no error)"=w310, "values"=w305, "starting address"=u16 4608, "MB session in"=w311) -> ("error out"=w315:errorcluster, "MB session out"=w316:refnum<class "MB_Master.lvclass">)  [unwired: 6 in]
      }
      frame "盲样测试" {
        n148 = Variant To Data(type=u8 0, Variant=w324) -> (data=w317:u8)  [unwired: 1 in, 1 out]
        n149 = property class="MB_Master"(reference=w323, error in=w320, "Properties:Slave ID"=w317) -> (reference out=w322:refnum<class "MB_Master.lvclass">, error out=w321:errorcluster)
        n150 = case shown="默认" w317 {
          tunnel: [u16[] [] ("values") u16[] [33539, 0] ("values") u16[] [23555, 0] ("values")] -> w319
          frame Default {
          }
          frame 1 {
            # "总磷盲样测试命令"
          }
          frame 3 {
            # "氨氮盲样测试"
          }
        }
        n151 = call <vilib>:"Write Multiple Registers.vi"("error in (no error)"=w321, "values"=w319, "starting address"=u16 24592, "MB session in"=w322) -> ("error out"=w326:errorcluster, "MB session out"=w327:refnum<class "MB_Master.lvclass">)  [unwired: 6 in]
      }
      frame "debug" {
        n152 = Variant To Data(type=cluster{"站号":u16, "控制命令":u16[]} {"站号"=0, "控制命令"=[]} ("输出簇"), Variant=w341) -> (data=w335:cluster{"站号":u16, "控制命令":u16[]})  [unwired: 1 in, 1 out]
        n153 = Unbundle By Name(w335) -> ("站号"=w331:u16, "控制命令"=w333:u16[])
        n154 = property class="MB_Master"(reference=w340, error in=w337, "Properties:Slave ID"=w331) -> (reference out=w339:refnum<class "MB_Master.lvclass">, error out=w338:errorcluster)
        n155 = Index Array(array=w333) -> (element=w334:u16)  [unwired: 1 in]
        n156 = global write "VAR总磷总氮全局变量.vi" "控制命令"(w334) -> ()
        n157 = call <vilib>:"Write Multiple Registers.vi"("error in (no error)"=w338, "values"=w333, "starting address"=u16 24594, "MB session in"=w339) -> ("error out"=w342:errorcluster, "MB session out"=w343:refnum<class "MB_Master.lvclass">)  [unwired: 6 in]
      }
      frame "读测量数据区" {
        n158 = Variant To Data(type=u8 1 ("Slave ID"), Variant=w358) -> (data=w345:u8)  [unwired: 1 in, 1 out]
        n159 = property class="MB_Master"(reference=w357, error in=w355, "Properties:Slave ID"=w345) -> (reference out=w356:refnum<class "MB_Master.lvclass">, error out=w354:errorcluster)
        n160 = global read "VAR总磷总氮全局变量.vi" "测量数据区数组"() -> (w351:T5)
        n161 = call <vilib>:"Read Holding Registers.vi"("error in (no error)"=w354, "quantity"=u16 105, "starting address"=u16 4096, "MB session in"=w356) -> ("error out"=w363:errorcluster, "Registers"=w353:u16[], "MB session out"=w362:refnum<class "MB_Master.lvclass">)  [unwired: 5 in]
        n162 = call "id参数转换.vi"("id"=w345) -> ("数组资源索引"=w344:i32)  [unwired: 9 in, 1 out]
        n163 = call "测量数据区.vi"("数组"=w353) -> ("测量数据区"=w350:T2)  [unwired: 10 in]
        "测量数据区" <- w350
        n164 = Index Array(array=w351, index #1=w344, index #2=1 ("索引")) -> (element #1=w352:T2, element #2=w346:T2)
        n165 = global write "VAR总磷总氮全局变量.vi" "测量数据区"(w350) -> ()
        n166 = case shown="1" w345 {
          tunnel: w350 -> [w364 w365 w385 w387 w389]
          tunnel: w353 -> [_ w374 w386 w388 w390]
          tunnel: w352 -> [_ w367 _ _ _]
          tunnel: [w364 w369 w385 w387 w389] -> w349
          tunnel: w346 -> [_ w366 _ _ _]
          frame 0, Default {
          }
          frame 1 {
            n167 = global read "VAR总磷总氮全局变量.vi" "模块名称"() -> (w373:string)
            n168 = Search and Replace String(input string=w373, search string="总磷" ("搜索字符串")) -> (result string=w370:string, offset past replacement=w371:i32)  [unwired: 6 in, 2 out]
            n169 = case shown="默认" w371 {
              tunnel: w370 -> [_ w379]
              tunnel: [_ w375] -> w368
              frame -1 {
              }
              frame Default {
                n170 = Search and Replace String(input string=w379, search string="总氮" ("搜索字符串")) -> (offset past replacement=w377:i32)  [unwired: 6 in, 3 out]
                n171 = Not Equal?(x=w377, y=-1) -> (x != y?=w375:bool)
              }
            }
            n172 = case shown="真" w368 {
              tunnel: [w380 w384] -> w369
              tunnel: w367 -> [_ w383]
              tunnel: w366 -> [_ w382]
              tunnel: w365 -> [w380 w381]
              frame False {
              }
              frame True {
                # "启动总氮时间自动对齐"
                n173 = call "数据时间对齐.vi"("待对齐时间"=w381, "对齐参考时间"=w382, "已对齐时间输入"=w383) -> ("已对齐时间输出"=w384:T2)  [unwired: 8 in]
              }
            }
            "总磷测量数据区" <- w374
          }
          frame 2 {
            "总氮测量数据区" <- w386
          }
          frame 3 {
            "氨氮测量数据区" <- w388
          }
          frame 22 {
            "COD测量数据区" <- w390
          }
        }
        n174 = Replace Array Subset(array=w351, new element=w349, index=w344) -> (w348:T5)
        n175 = global write "VAR总磷总氮全局变量.vi" "测量数据区数组"(w348) -> ()
      }
      frame "读状态告警区" {
        n176 = Variant To Data(type=u8 1 ("Slave ID"), Variant=w399) -> (data=w392:u8)  [unwired: 1 in, 1 out]
        n177 = property class="MB_Master"(reference=w402, error in=w403, "Properties:Slave ID"=w392) -> (reference out=w401:refnum<class "MB_Master.lvclass">, error out=w400:errorcluster)
        n178 = call "id参数转换.vi"("id"=w392) -> ("数组资源索引"=w391:i32)  [unwired: 9 in, 1 out]
        n179 = call <vilib>:"Read Holding Registers.vi"("error in (no error)"=w400, "quantity"=u16 29, "starting address"=u16 4224, "MB session in"=w401) -> ("error out"=w398:errorcluster, "Registers"=w396:u16[], "MB session out"=w407:refnum<class "MB_Master.lvclass">)  [unwired: 5 in]
        n180 = global read "VAR总磷总氮全局变量.vi" "状态告警区数组"() -> (w395:T7)
        n181 = call "状态告警区.vi"("数组"=w396) -> ("状态告警区"=w394:T4)  [unwired: 10 in]
        "状态告警区" <- w394
        n182 = global write "VAR总磷总氮全局变量.vi" "状态告警区"(w394) -> ()
        n183 = Unbundle By Name(w394) -> ("id"=w397:u16)
        n184 = Replace Array Subset(array=w395, new element=w394, index=w391) -> (w393:T7)
        n185 = case shown="22" w397 {
          tunnel: w394 -> [_ _ _ _ _]
          tunnel: w396 -> [_ w408 w409 w410 w411]
          frame 0, Default {
          }
          frame 1, 131 {
            "总磷状态告警区" <- w408
          }
          frame 2, 76 {
            "总氮状态告警区" <- w409
          }
          frame 3 {
            "氨氮状态告警区" <- w410
          }
          frame 22 {
            "COD状态告警区" <- w411
          }
        }
        n186 = global write "VAR总磷总氮全局变量.vi" "状态告警区数组"(w393) -> ()
      }
      frame "读关键参数区" {
        n187 = Variant To Data(type=u8 1 ("Slave ID"), Variant=w419) -> (data=w413:u8)  [unwired: 1 in, 1 out]
        n188 = property class="MB_Master"(reference=w422, error in=w423, "Properties:Slave ID"=w413) -> (reference out=w421:refnum<class "MB_Master.lvclass">, error out=w420:errorcluster)
        n189 = call "id参数转换.vi"("id"=w413) -> ("数组资源索引"=w412:i32)  [unwired: 9 in, 1 out]
        n190 = call <vilib>:"Read Holding Registers.vi"("error in (no error)"=w420, "quantity"=u16 19, "starting address"=u16 4256, "MB session in"=w421) -> ("error out"=w427:errorcluster, "Registers"=w417:u16[], "MB session out"=w426:refnum<class "MB_Master.lvclass">)  [unwired: 5 in]
        n191 = global read "VAR总磷总氮全局变量.vi" "关键参数区数组"() -> (w416:T6)
        n192 = call "关键参数区.vi"("数组"=w417) -> ("关键参数区"=w415:T3)  [unwired: 10 in]
        "关键参数区" <- w415
        n193 = global write "VAR总磷总氮全局变量.vi" "关键参数区"(w415) -> ()
        n194 = Replace Array Subset(array=w416, new element=w415, index=w412) -> (w414:T6)
        n195 = global write "VAR总磷总氮全局变量.vi" "关键参数区数组"(w414) -> ()
      }
      frame "shutdown" {
        n196 = call-dynamic "Close Session.vi"("error in (no error)"=w430, "MB session in"=w428) -> ("error out"=w429:errorcluster)  [unwired: 9 in]
        n197 = Flush Queue(queue=w432) -> (queue out=w431:refnum<queue>)  [unwired: 1 in, 2 out]
        n198 = Release Queue(queue=w431) -> ()  [unwired: 2 in, 3 out]
      }
    }
    n199 = global write "VAR总磷总氮全局变量.vi" "MB session in"(w270) -> ()
    n200 = Unbundle By Name(w278) -> ("status"=w274:bool)
    n201 = Not(x=w274) -> (.not. x?=w277:bool)
    "status" <- w277
    n202 = call <vilib>:"Boolean Crossing PtByPt.vi"("direction"=enum16{"either", "false-true", "true-false"}."false-true", "input"=w274) -> ("crossing"=w273:bool)  [unwired: 1 in]
    n203 = call "id参数转换.vi"("id"=w271) -> ("table输出"=w275:string)  [unwired: 9 in, 1 out]
    n204 = case shown="真" w273 {
      tunnel: w275 -> [_ w290]
      frame False {
      }
      frame True {
        n205 = Get Date/Time In Seconds() -> (seconds since 1Jan1904=w289:timestamp)
        n206 = Bundle By Name(cluster=T10 {"时间标识"=timestamp(0 s since 1904-01-01), "设备"="", "日志信息"="", "备注"=""} ("data in"), "时间标识"=w289, "设备"=w290, "日志信息"="通讯告警") -> (w288:T10)
        n207 = call "总磷总氮报警信息.vi"("data in"=w288) -> ()  [unwired: 10 in, 1 out]
      }
    }
    n208 = global write "VAR总磷总氮全局变量.vi" "通讯状态"(w277) -> ()
  }
